vi "Lorentz fit dispersive.vi"(10 "Y subset":dbl[](array[numeric]), 11 "X subset":dbl[](array[numeric])) -> (0 "error out":errorcluster, 1 "Initial params":dbl[](array[numeric]), 2 "best fit parameters":dbl[](array[numeric]), 3 "best nonlinear fit":dbl[](array[numeric]), 4 "residue":dbl)   [LabVIEW 2015]
uses:
  <vilib>/gmath/NumericalOptimization/Nonlinear Curve Fit LM bound.vi
  <vilib>/gmath/NI_Gmath.lvlib
panel:
  # "Fitting to a dispersive Lorentzian-like function\n(called \"lfun3c_dispersive\" in my Matlab functions):\nF = p1.*(x-p2)./((x-p2).^2+(p3^2)) + p4"
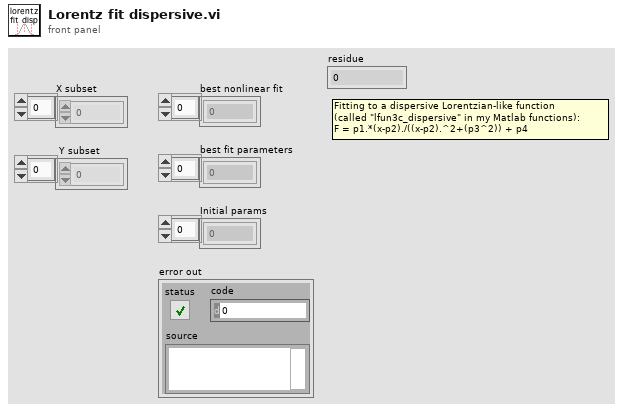
[diagram p1: front panel]
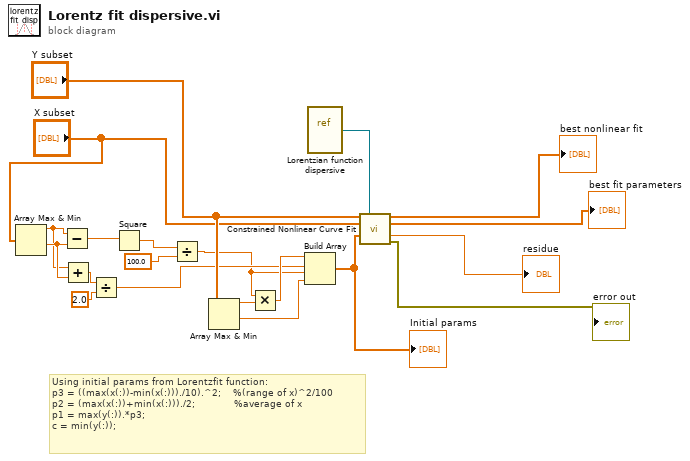
[diagram p0: block diagram]
diagram:
  # "Using initial params from Lorentzfit function:\np3 = ((max(x(:))-min(x(:)))./10).^2;    %(range of x)^2/100\np2 = (max(x(:))+min(x(:)))./2;             %average of x\np1 = max(y(:)).*p3;\nc = min(y(:));"
  n1 = Array Max & Min(array="X subset") -> (max value=w3:dbl, min value=w7:dbl)  [unwired: 2 out]
  n2 = Subtract(x=w3, y=w7) -> (x-y=w8:dbl)
  n3 = Add(x=w3, y=w7) -> (x+y=w6:dbl)
  n4 = Divide(x=w6, y=2.0) -> (x/y=w2:dbl)
  n5 = Square(x=w8) -> (x^2=w10:dbl)
  n6 = Divide(x=w10, y=100.0) -> (x/y=w1:dbl)
  n7 = Array Max & Min(array="Y subset") -> (max value=w14:dbl, min value=w13:dbl)  [unwired: 2 out]
  n8 = Multiply(x=w1, y=w14) -> (x*y=w11:dbl)
  n9 = Build Array(w11, w2, w1, w13) -> (w16:dbl[])
  "Initial params" <- w16
  n10 = vi-ref "Lorentzian function dispersive.vi"() -> (w20:refnum<vi>)
  n11 = call-poly <vilib>:"Constrained Nonlinear Curve Fit.vi"("Y"="Y subset", "f(x,a)"=w20, "X"="X subset", "initial parameters"=w16) -> ("best nonlinear fit"=→"best nonlinear fit":dbl[], "best fit parameters"=→"best fit parameters":dbl[], "residue"=→"residue":dbl, "error out"=→"error out":errorcluster)  [unwired: 6 in, 2 out]
